vi "___2ddata_to_multigraph.vi"(4 "列":i32[](array[numeric]), 7 "データ配列":dbl[][](array[numeric])) -> (3 "XYグラフ":cluster{"データ配列":dbl[], "データ配列":dbl[]}[](graph))   [LabVIEW 2017]
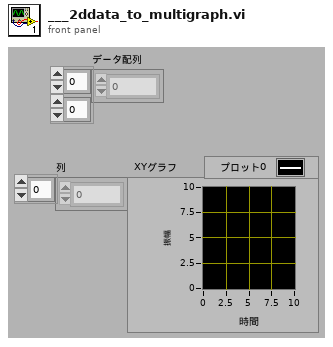
[diagram p1: front panel]
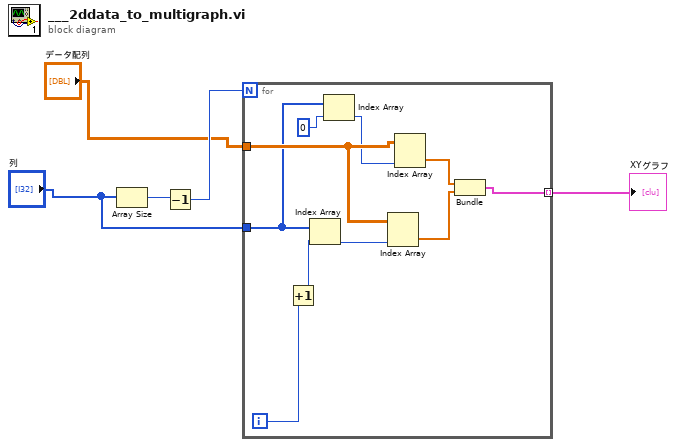
[diagram p0: block diagram]
diagram:
  n1 = Array Size(array="列") -> (size(s)=w5:i32)
  n2 = Decrement(x=w5) -> (x-1=w4:i32)
  n3 = for {
    N: w4 -> [_]
    tunnel: "列" -> [w11]
    tunnel: "データ配列" -> [w13]
    tunnel: [w6] -> w1 mode=indexing
    i -> [w15]
    n4 = Increment(x=w15) -> (x+1=w9:i32)
    n5 = Index Array(array=w11, index=w9) -> (element=w14:i32)
    n6 = Index Array(array=w11, index=0) -> (element=w12:i32)
    n7 = Index Array(array=w13, index (col)=w14) -> (element=w7:dbl[])  [unwired: 1 in]
    n8 = Index Array(array=w13, index (col)=w12) -> (element=w8:dbl[])  [unwired: 1 in]
    n9 = Bundle("データ配列"=w8, "データ配列"=w7) -> (w6:cluster{"データ配列":dbl[], "データ配列":dbl[]})  [unwired: 1 in]
  }
  "XYグラフ" <- w1
